vi "user32_EmptyClipboard.vi"(8 "错误输入（无错误）":errorcluster) -> (0 "错误输出":errorcluster, 3 "success?":bool)   [LabVIEW 2011]
doc: "该函数清空剪切板并释放剪切板内数据的句柄。函数在之后会将剪切板的所有权指派给当前打开剪切板的窗口。"
uses:
  user32.dll
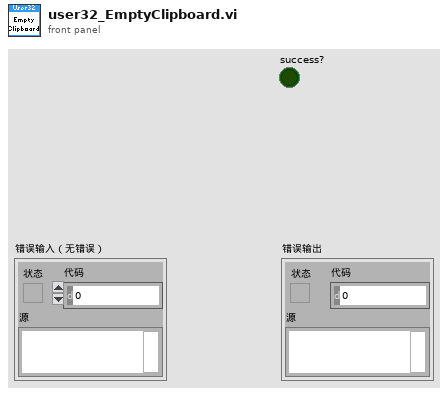
[diagram p1: front panel]
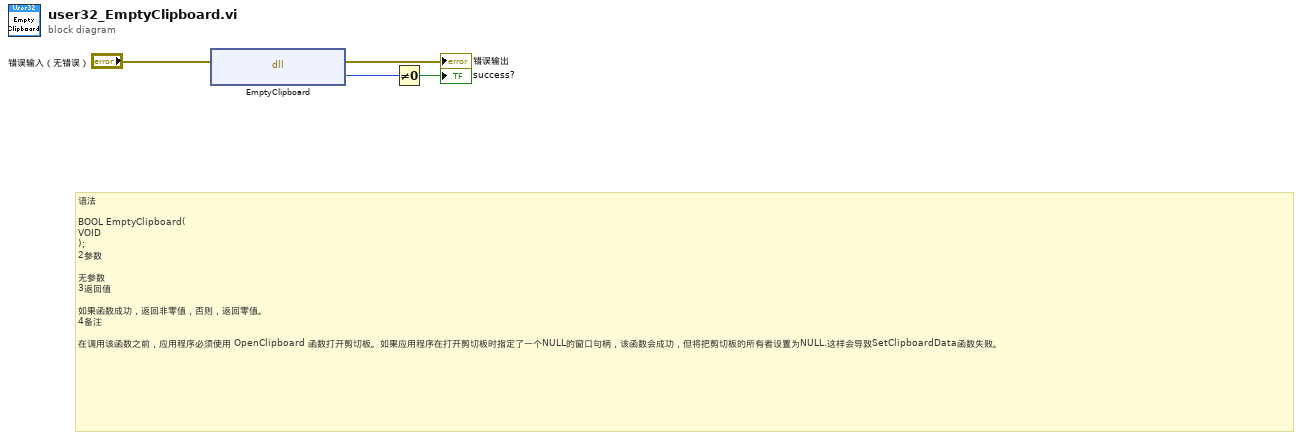
[diagram p0: block diagram]
diagram:
  # "语法\n\nBOOL EmptyClipboard(\nVOID\n);\n2参数\n\n无参数\n3返回值\n\n如果函数成功，返回非零值，否则，返回零值。\n4备注\n\n在调用该函数之前，应用程序必须使用 OpenClipboard 函数打开剪切板。如果应用程序在打开剪切板时指定了一个NULL的窗口句柄，该函数会成功，但将把剪切板的所有者设置为NULL.这样会导致SetClipboardData函数失败。"
  n1 = dll-call lib="user32.dll" fn="EmptyClipboard"(error in="错误输入（无错误）") -> (error out=→"错误输出":errorcluster, "Bool"=w2:u8)  [unwired: 2 in, 1 out]
  n2 = Not Equal To 0?(x=w2) -> (x != 0?=→"success?":bool)
